vi "Launch OOQMH.vi"(8 "error in (no error)":errorcluster, 11 "OOQMH in":refnum<class "OOQMH.lvclass">) -> (0 "error out":errorcluster, 2 "Message Queue":refnum<queue>)   [LabVIEW 2024, in "OOQMH.lvlib" / "OOQMH.lvclass"]
uses:
  OOQMH.lvclass
  Message/Message.lvclass
  OOQMH.vi
  OOQMH.lvclass/OOQMH.ctl
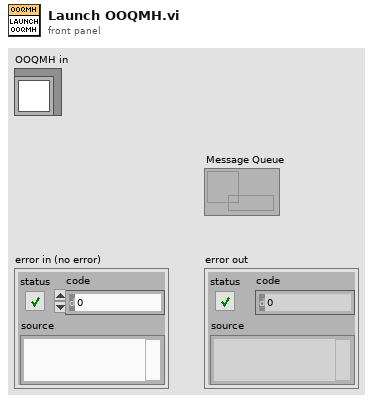
[diagram p1: front panel]
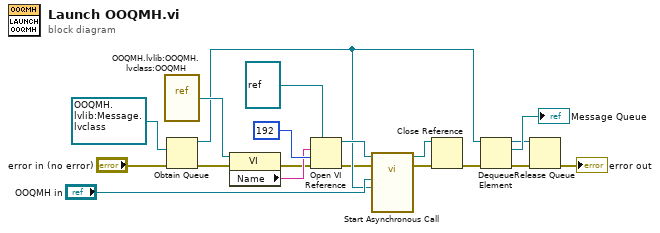
[diagram p0: block diagram]
diagram:
  n1 = vi-ref "OOQMH.lvlib:OOQMH.lvclass:OOQMH.vi"() -> (w12:refnum<vi>)
  n2 = Obtain Queue(element data type=refnum<queue> refnum ("Message Queue"), error in (no error)="error in (no error)") -> (queue out=w10:refnum<queue>, error out=w7:errorcluster)  [unwired: 3 in, 1 out]
  n3 = property class="VI"(reference=w12, error in=w7) -> (error out=w6:errorcluster, "Name"=w11:string)  [unwired: 1 out]
  n4 = Open VI Reference(type specifier VI Refnum (for type only)=refnum<vi> refnum, vi path=w11, options=192, error in (no error)=w6) -> (vi reference=w18:refnum<vi>, error out=w5:errorcluster)  [unwired: 2 in]
  n5 = call-by-ref "Start Asynchronous Call"(reference=w18, error in=w5, "Sharing Queue"=w10, "OOQMH in"="OOQMH in") -> (reference out=w14:refnum<vi>, error out=w13:errorcluster)  [unwired: 10 in]
  n6 = Close Reference(reference=w14, error in (no error)=w13) -> (error out=w9:errorcluster)
  n7 = Dequeue Element(queue=w10, error in (no error)=w9) -> (queue out=w2:refnum<queue>, element=→"Message Queue":refnum<queue>, error out=w3:errorcluster)  [unwired: 1 in, 1 out]
  n8 = Release Queue(queue=w2, error in (no error)=w3) -> (error out=→"error out":errorcluster)  [unwired: 1 in, 2 out]
